vi "Pause Unpause.vi"(8 "error in":errorcluster, 11 "PauseUnpause Ref":refnum<vi>) -> (0 "error out":errorcluster, 3 "New Data":string[][](array[string]))   [LabVIEW 2025, in "Automotive Ethernet Bus Monitor UI.lvlib"]
doc: "Returning the new captured data when unpaused. During pause and error returns an empty array."
uses:
  Automotive Ethernet Bus Monitor UI.lvlib
  Table Buffer/Dequeue Data.vi
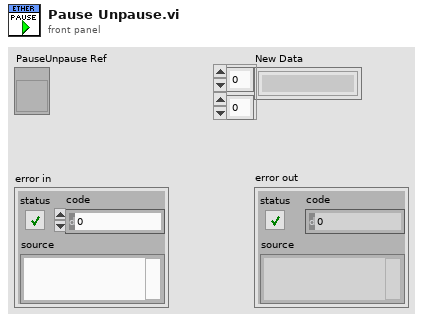
[diagram p1: front panel]
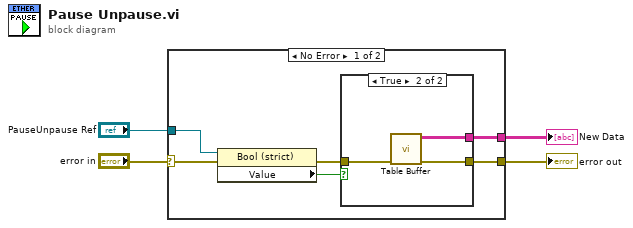
[diagram p0: block diagram]
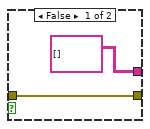
[diagram p2: hidden frame]
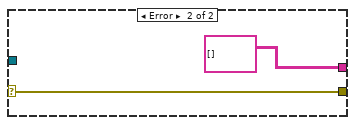
[diagram p3: hidden frame]
diagram:
  n1 = case shown="No Error" "error in" {
    selector: "error in" -> [w5 w17]
    tunnel: [w10 string[][] [] ("Dataframe 3")] -> w4
    tunnel: "PauseUnpause Ref" -> [w7 _]
    tunnel: [w6 w17] -> w2
    frame No Error {
      n2 = property class="Bool (strict)"(reference=w7, error in=w5) -> (error out=w9:errorcluster, "Value"=w8:bool)  [unwired: 1 out]
      n3 = case shown="True" w8 {
        tunnel: w9 -> [w11 w15]
        tunnel: [string[][] [] ("Dataframe 3") w14] -> w10
        tunnel: [w11 w13] -> w6
        frame False {
        }
        frame True {
          n4 = call-poly "Table Buffer.vi"("error in"=w15) -> ("error out"=w13:errorcluster, "Data"=w14:string[][])  [unwired: 9 in]
        }
      }
    }
    frame Error {
    }
  }
  "New Data" <- w4
  "error out" <- w2
